vi "acquire cursor window data - no plot.vi"(9 "z in":cdb[](array[numeric]), 10 "omega in":dbl[](array[numeric]), 11 "cursor window in":T1={"left"=2378.60310421286, "right "=2421.6740576496672, "center"=2421.6740576496672, "window"=2421.6740576496672, "skew"=2421.6740576496672, "default window frac"=2421.6740576496672, "kind"=enum."skewed", "skew.left"=2421.6740576496672, "skew.right"=2421.6740576496672, "wing order"=enum."back"}) -> (1 "z out":cdb[](array[numeric]), 2 "omega  out":dbl[](array[numeric]))   [LabVIEW 2010]
uses:
  cursor winow control -- no plot.ctl
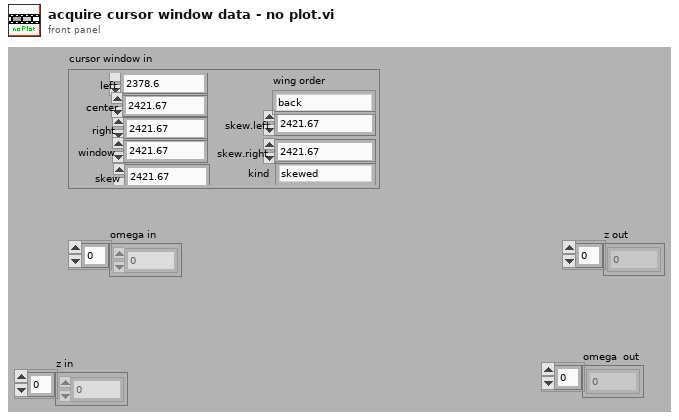
[diagram p1: front panel]
types:
  T1 = typedef "cursor winow control -- no plot.ctl" = cluster{"left":dbl, "right ":dbl, "center":dbl, "window":dbl, "skew":dbl, "default window frac":dbl, "kind":enum16{"symmetric", "skewed", "fancy"}, "skew.left":dbl, "skew.right":dbl, "wing order":enum16{"forw", "back"}}
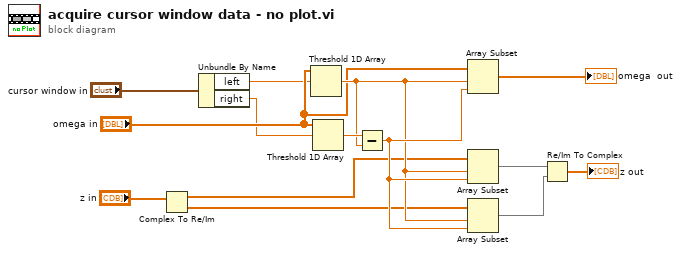
[diagram p0: block diagram]
diagram:
  n1 = Complex To Re/Im(x + iy="z in") -> (x=w7:dbl[], y=w6:dbl[])
  n2 = Unbundle By Name("cursor window in") -> ("left"=w2:dbl, "right"=w3:dbl)
  n3 = Threshold 1D Array(2:w2, 3:"omega in") -> (0:w12:dbl)  [unwired: 1 in]
  n4 = Threshold 1D Array(2:w3, 3:"omega in") -> (0:w14:dbl)  [unwired: 1 in]
  n5 = Subtract(x=w14, y=w12) -> (x-y=w13:dbl)
  n6 = Array Subset(array="omega in", index=w12, length=w13) -> (→"omega  out":dbl[])
  n7 = Array Subset(array=w7, index=w12, length=w13) -> (w10:dbl[])
  n8 = Array Subset(array=w6, index=w12, length=w13) -> (w11:dbl[])
  n9 = Re/Im To Complex(1:w11, 2:w10) -> (0:→"z out":cdb[])
